vi "SetAlignment.vi"(8 "error":errorcluster caption="错误输入（无错误）", 9 "Vertical Alignment(垂直)":enum16{"xlTop", "xlCenter", "xlBottom"}(ring), 10 "Horizontal Alignment(水平)":enum16{"xlRight", "xlLeft", "xlCenter"}(ring), 11 "Excel._Worksheet":refnum<k7>) -> (0 "error out":errorcluster caption="错误输出", 3 "Excel._Worksheet":refnum<k7>)   [LabVIEW 2014]
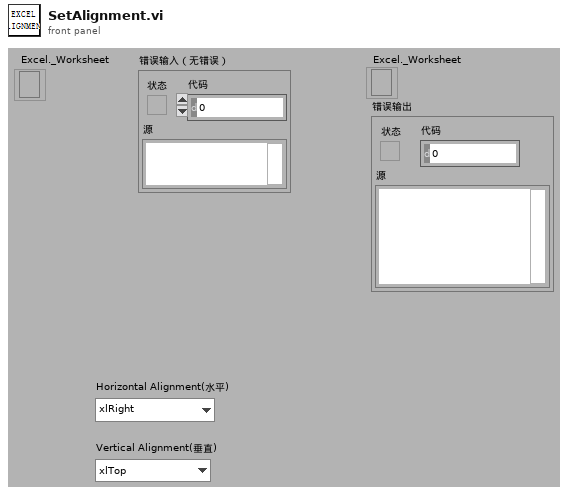
[diagram p1: front panel]
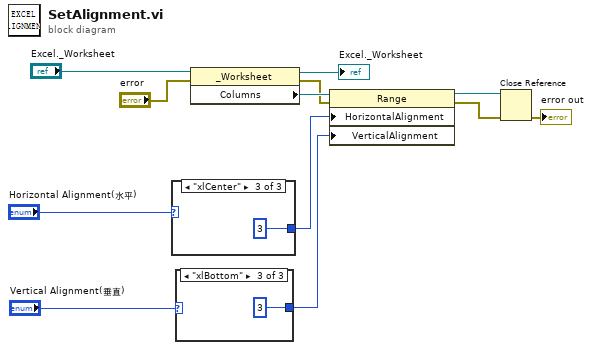
[diagram p0: block diagram]
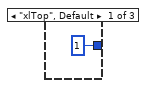
[diagram p2: hidden frame]
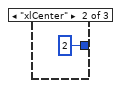
[diagram p3: hidden frame]
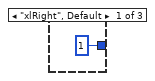
[diagram p4: hidden frame]
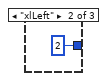
[diagram p5: hidden frame]
diagram:
  n1 = case shown="\"xlCenter\"" "Horizontal Alignment(水平)" {
    tunnel: [1 2 3] -> w7
    frame "xlRight", Default {
    }
    frame "xlLeft" {
    }
    frame "xlCenter" {
    }
  }
  n2 = case shown="\"xlBottom\"" "Vertical Alignment(垂直)" {
    tunnel: [1 2 3] -> w6
    frame "xlTop", Default {
    }
    frame "xlCenter" {
    }
    frame "xlBottom" {
    }
  }
  n3 = property class="_Worksheet"(reference="Excel._Worksheet", error in="error") -> (reference out=→"Excel._Worksheet":refnum<k7>, error out=w1:errorcluster, "Columns"=w3:refnum<k7>)
  n4 = property class="Range"(reference=w3, error in=w1, "HorizontalAlignment"=w7, "VerticalAlignment"=w6) -> (reference out=w12:refnum<k7>, error out=w11:errorcluster)
  n5 = Close Reference(reference=w12, error in (no error)=w11) -> (error out=→"error out":errorcluster)
